vi "Create Channel Config.vi"(0 "Name":string, 1 "Data Type":T1=enum."int32", 2 "Component":string, 3 "Units":string, 4 "Description":string, 5 "Bit Field Elements":T3[](array[typedef]), 7 "Enum Types":T4[](array[typedef])) -> (16 "Output":T2={"name"="", "data_type"=enum."int32", "description"="", "component"="", "unit"="", "bit_field_elements"=[], "enum_types"=[]})   [LabVIEW 2024, in "Sift Client.lvlib"]
doc: "Create a Channel Config object."
uses:
  Sift Client.lvlib
  Private/Typedefs/Ingestion Config/Channel Config.ctl
  Types/Data Type.ctl
  Types/Bit Field.ctl
  Types/Enum.ctl
panel:
  in  "Channel Config":T2={"name"="", "data_type"=enum."int32", "description"="", "component"="", "unit"="", "bit_field_elements"=[], "enum_types"=[]}
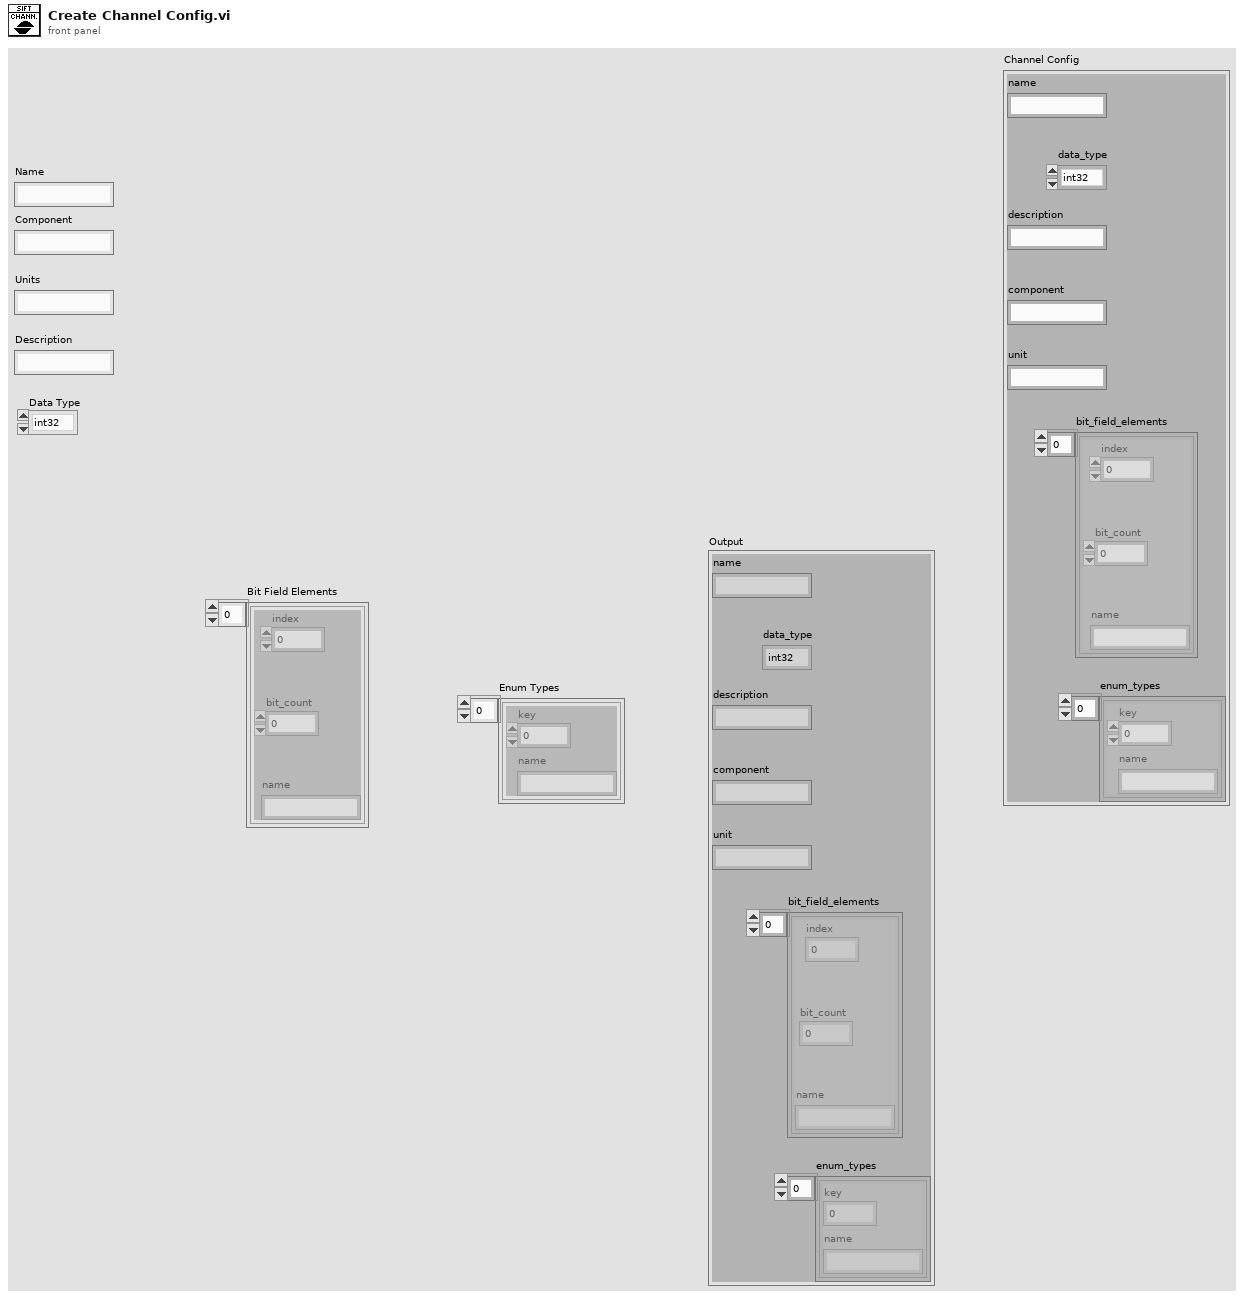
[diagram p1: front panel]
types:
  T1 = typedef "Sift Client.lvlib/Data Type.ctl" = enum8{"double", "float", "uint64", "int64", "uint32", "int32", "bool", "enum", "string"}
  T2 = typedef "Sift Client.lvlib/Channel Config.ctl" = cluster{"name":string, "data_type":T1, "description":string, "component":string, "unit":string, "bit_field_elements":T3[], "enum_types":T4[]}
  T3 = typedef "Bit Field.ctl" = cluster{"index":u32, "bit_count":u32, "name":string}
  T4 = typedef "Sift Client.lvlib/Enum.ctl" = cluster{"key":u32, "name":string}
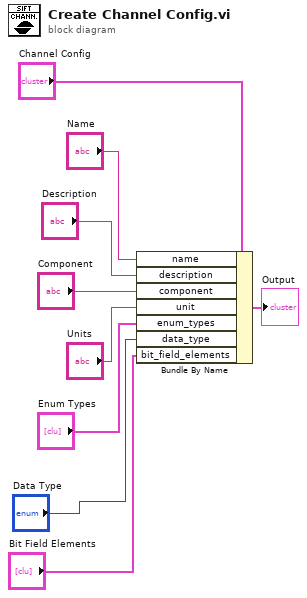
[diagram p0: block diagram]
diagram:
  n1 = Bundle By Name(cluster="Channel Config", "name"="Name", "description"="Description", "component"="Component", "unit"="Units", "enum_types"="Enum Types", "data_type"="Data Type", "bit_field_elements"="Bit Field Elements") -> (→"Output":T2)
